vi "File List Get Count.vi"(11 "File List in":refnum<class "File List.lvclass">) -> (2 "Count":i32, 3 "File List out":refnum<class "File List.lvclass">)   [LabVIEW 2011, in "COSYLib.lvlib" / "File List.lvclass"]
uses:
  File List.lvclass
  File List.lvclass/File List.ctl
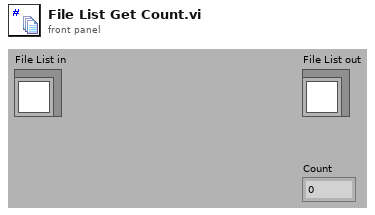
[diagram p1: front panel]
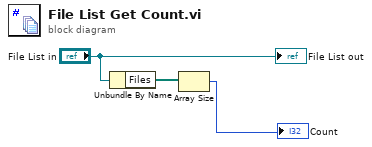
[diagram p0: block diagram]
diagram:
  n1 = Unbundle By Name("File List in") -> ("Files"=w3:path[])
  n2 = Array Size(array=w3) -> (size(s)=→"Count":i32)
  "File List out" <- "File List in"
